vi "aft_AFT_Linear_Prediction_Data_Type_Matching_Sub.vi"(11 "adaptive filter in":refnum<k20>) -> (3 "error":i32)   [LabVIEW 2017, in "NI_AdaptiveFilter.lvlib"]
uses:
  <vilib>/addons/Adaptive Filters/NI_AdaptiveFilter.lvlib
  <resource>/AdaptiveFilters.dll
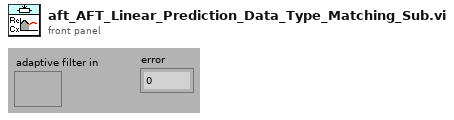
[diagram p1: front panel]
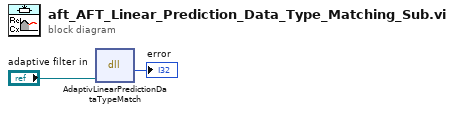
[diagram p0: block diagram]
diagram:
  n1 = dll-call lib="C:/Program Files/National Instruments/LabVIEW 2017/resource/AdaptiveFilters.dll" fn="AdaptivLinearPredictionDataTypeMatch" ("Complex Data Initialization")("pSession"="adaptive filter in") -> ("err"=→"error":i32)  [unwired: 4 in, 2 out]
